vi "NotifierReader.vi"() -> (2 "NumericOut":i32)   [LabVIEW 2014]
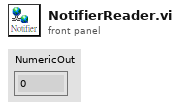
[diagram p1: front panel]
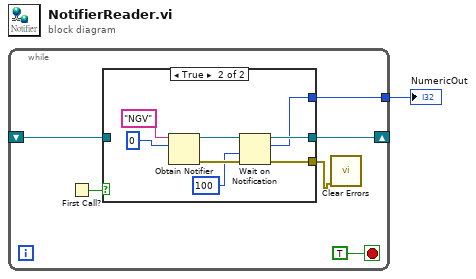
[diagram p0: block diagram]
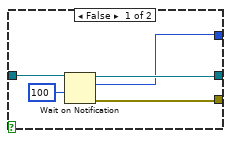
[diagram p2: hidden frame]
diagram:
  n1 = while {
    shift-right: [w5] -> _
    shift-left: _ -> [w4]
    tunnel: [w3] -> w1
    stop <- TRUE stop-if-true
    n2 = First Call?() -> (First Call?: T/F=w7:bool)
    n3 = case shown="True" w7 {
      tunnel: [w11 w16] -> w5
      tunnel: w4 -> [w12 _]
      tunnel: [w10 w15] -> w3
      tunnel: [w9 w14] -> w2
      frame False {
        n4 = Wait on Notification(notifier=w12, timeout in ms (-1)=100) -> (notifier out=w11:refnum<notifier>, notification=w10:i32, error out=w9:errorcluster)  [unwired: 2 in, 1 out]
      }
      frame True {
        n5 = Obtain Notifier(name (unnamed)="NGV", notification data type=0 ("Numeric")) -> (notifier out=w17:refnum<notifier>, error out=w18:errorcluster)  [unwired: 2 in, 1 out]
        n6 = Wait on Notification(notifier=w17, timeout in ms (-1)=100, error in (no error)=w18) -> (notifier out=w16:refnum<notifier>, notification=w15:i32, error out=w14:errorcluster)  [unwired: 1 in, 1 out]
      }
    }
    n7 = call <vilib>:"Clear Errors.vi"("error in (no error)"=w2) -> ()  [unwired: 5 in, 2 out]
  }
  "NumericOut" <- w1
